vi "GEA2_Reregister.vi"(0 "Event Registration Refnum":refnum<event-registration>, 5 "Board Index":i32 min=0 max=10 step=1, 11 "Error In":errorcluster) -> (4 "GEA2 Reference Out":refnum<k24>, 6 "Board ID":string, 8 "Event Registration Refnum 2":refnum<event-registration>, 15 "Error Out":errorcluster)   [LabVIEW 2023]
uses:
  D:/Common/LabVIEW GEA2 Toolkit/source/GEA3 DLL Source/GeaCommunication.dll
  Common/LabVIEW GEA2 Toolkit/source/GEA3 DLL Source/GeaCommunication.dll
  Common/LabVIEW GEA2 Toolkit/GEA3/type defs/Data Out.ctl
  Common/LabVIEW GEA2 Toolkit/GEA3/advanced/GEA2 Message Received Event Handler.vi
  Common/LabVIEW GEA2 Toolkit/GEA3/advanced/GEA2 Message Sent Event Handler.vi
  Common/LabVIEW GEA2 Toolkit/GEA3/library/GEA2_Toolkit.lvlib
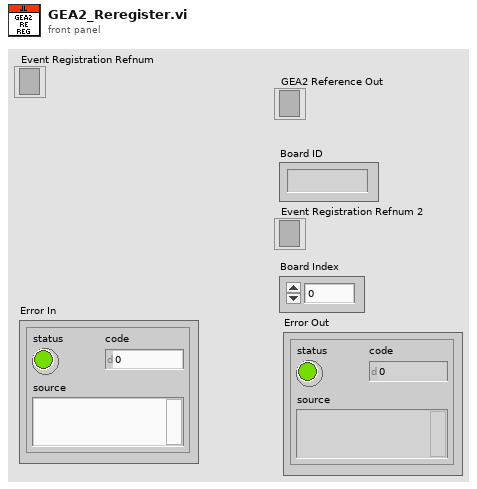
[diagram p1: front panel]
types:
  T1 = typedef "GEA2_Toolkit.lvlib/Data Out.ctl" = cluster{"Source":u8, "Destination":u8, "Command":u8, "Length":u8, "CRC":u16, "Message":string}
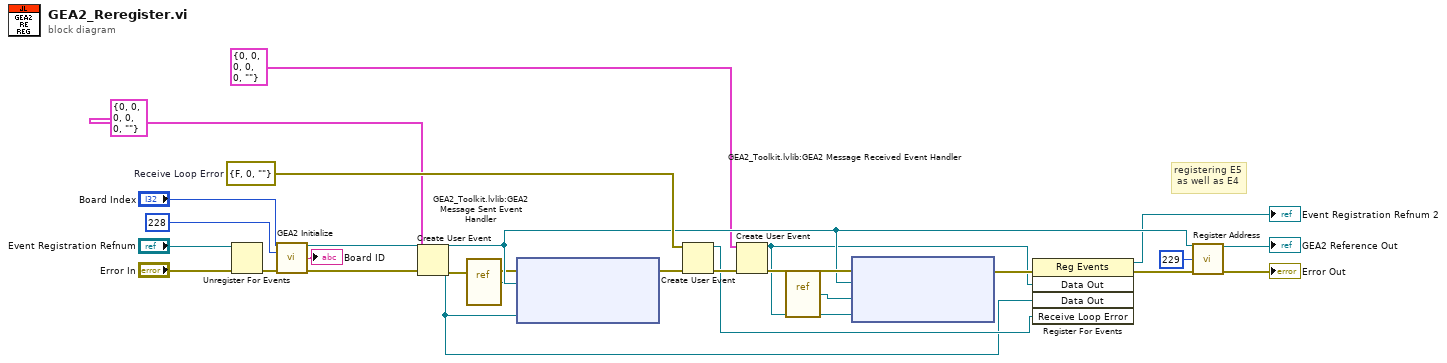
[diagram p0: block diagram]
diagram:
  w24 = errorcluster {"status"=FALSE, "code"=0, "source"=""}  # Receive Loop Error
  # "registering E5\n as well as E4"
  n1 = Unregister For Events(event registration refnum="Event Registration Refnum", error in="Error In") -> (error out=w20:errorcluster)
  n2 = call "GEA2 Initialize.vi"("Board Index"="Board Index", "Source Address"=u8 228, "error in"=w20) -> ("GEA2 Reference Out"=w12:refnum<k24>, "Board ID"=→"Board ID":string, "error out"=w13:errorcluster)  [unwired: 9 in, 1 out]
  n3 = Create User Event(user event datatype=T1 {"Source"=0, "Destination"=0, "Command"=0, "Length"=0, "CRC"=0, "Message"=""} ("Data Out"), error in=w13) -> (user event=w7:refnum<user-event>, error out=w11:errorcluster)
  n4 = vi-ref "GEA2_Toolkit.lvlib:GEA2 Message Sent Event Handler.vi"() -> ("vi reference"=w3:refnum<vi>)
  n5 = node(w11, w12, w3, w7) -> (w10:errorcluster)  [unwired: 1 in, 1 out]
  n6 = Create User Event(user event datatype=w24, error in=w10) -> (user event=w9:refnum<user-event>, error out=w23:errorcluster)
  n7 = Create User Event(user event datatype=T1 {"Source"=0, "Destination"=0, "Command"=0, "Length"=0, "CRC"=0, "Message"=""} ("Data Out"), error in=w23) -> (user event=w8:refnum<user-event>, error out=w21:errorcluster)
  n8 = vi-ref "GEA2_Toolkit.lvlib:GEA2 Message Received Event Handler.vi"() -> ("vi reference"=w4:refnum<vi>)
  n9 = node(w21, w12, w4, w8) -> (w22:errorcluster)  [unwired: 1 in, 1 out]
  n10 = register-events(error in=w22, w8, w7, w9) -> (reference out=→"Event Registration Refnum 2":refnum<event-registration>, error out=w17:errorcluster)  [unwired: 1 in]
  n11 = call "Register Address.vi"("GEA2 Reference In"=w12, "Address"=u8 229 ("Numeric Control"), "Error In"=w17) -> ("GEA2 Reference Out"=→"GEA2 Reference Out":refnum<k24>, "Error Out"=→"Error Out":errorcluster)  [unwired: 11 in]
